vi "G#RemoteProxy_Create.vi"(0 "reference in":refnum<class "G#RemoteProxy.lvclass">, 1 "proxy class ref":refnum<class "G#RemoteProxy.lvclass">, 2 "object name":string, 3 "class name":string, 4 "lvlib hierarchy":string[](array[string]), 5 "full class name":string, 6 "no registration (F)":bool, 7 "error in (no error)":errorcluster, 8 "create method":T3=enum."Create or look up existing", 9 "user counter (T)?":bool=TRUE, 10 "remote object ref":refnum<class "G#Object.lvclass">, 11 "class hierarchy":T2[](array[typedef]), 12 "connection ID":refnum<k5>, 13 "id":u32, 14 "address":u32, 15 "owner":string, 17 "in memory?":bool) -> (20 "reference out":refnum<class "G#RemoteProxy.lvclass">, 23 "# of users":i32, 27 "error out":errorcluster)   [LabVIEW 2017, in "G#RemoteProxy.lvclass"]
doc: "Constructor."
uses:
  <vilib>/addons/_AddQ/G#Debugger/G#RemoteProxy/G#RemoteProxy.lvclass
  C:/Program Files (x86)/National Instruments/LabVIEW 2017/vi.lib/addons/_AddQ/G#Object/G#Object.lvclass
  <vilib>/addons/_AddQ/G#Object/utils/G#Object_CreateMethod.ctl
  <vilib>/addons/_AddQ/G#Object/utils/G#Object_ClassHierarchy.ctl
  <vilib>/addons/_AddQ/G#Debugger/G#RemoteProxy/protected/ObjectAttributesProxy.ctl
  <vilib>/addons/_AddQ/G#Object/G#Object.lvclass
  <vilib>/addons/_AddQ/G#Debugger/G#RemoteProxy/G#RemoteProxy.lvclass/G#RemoteProxy.ctl
panel:
  in  "object attributes type":T1
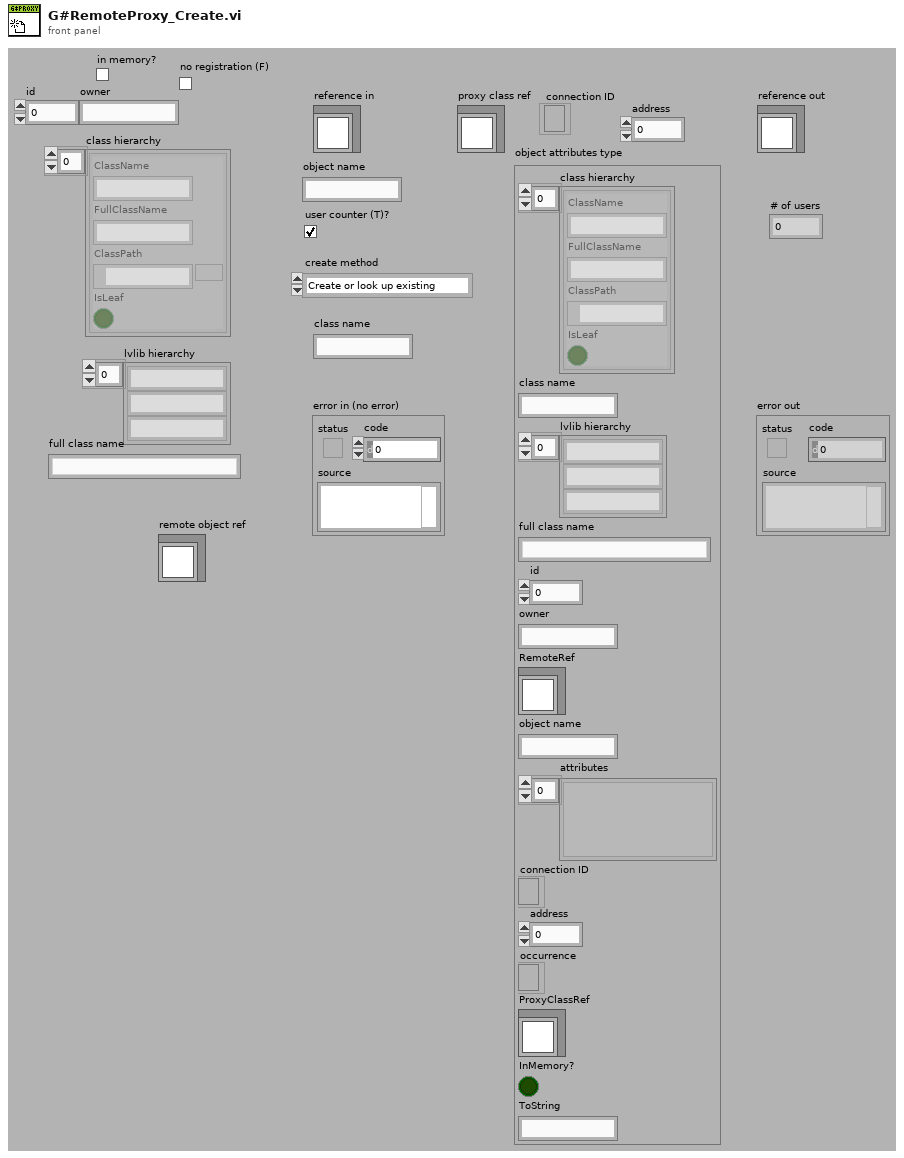
[diagram p1: front panel]
types:
  T1 = typedef "G#RemoteProxy.lvclass/ObjectAttributesProxy.ctl" = cluster{"class hierarchy":T2[], "class name":string, "lvlib hierarchy":string[], "full class name":string, "id":u32, "owner":string, "RemoteRef":refnum<class "G#Object.lvclass">, "object name":string, "attributes":variant[], "connection ID":refnum<k5>, "address":u32, "occurrence":refnum<k4>, "ProxyClassRef":refnum<class "G#RemoteProxy.lvclass">, "InMemory?":bool, "ToString":string}
  T2 = typedef "G#Object.lvclass/G#Object_ClassHierarchy.ctl" = cluster{"ClassName":string, "FullClassName":string, "ClassPath":path, "IsLeaf":bool}
  T3 = typedef "G#Object.lvclass/G#Object_CreateMethod.ctl" = enum16{"Create", "Create or look up existing", "Look up existing"}
  T4 = typedef "G#RemoteProxy.lvclass/ObjectAttributesRef.ctl" = refnum<data-value>
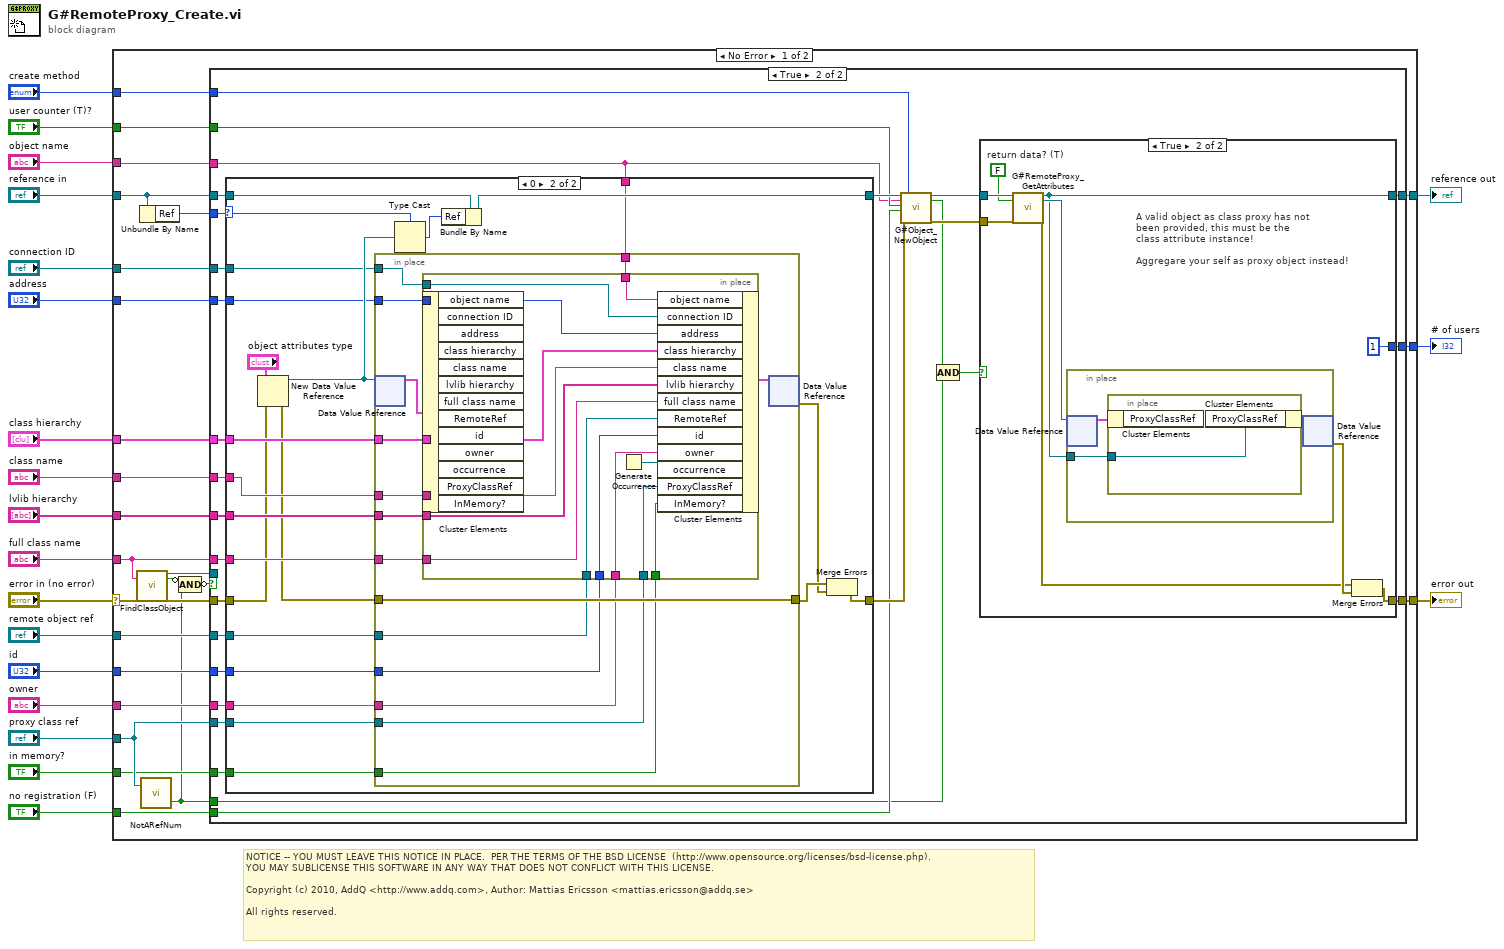
[diagram p0: block diagram]
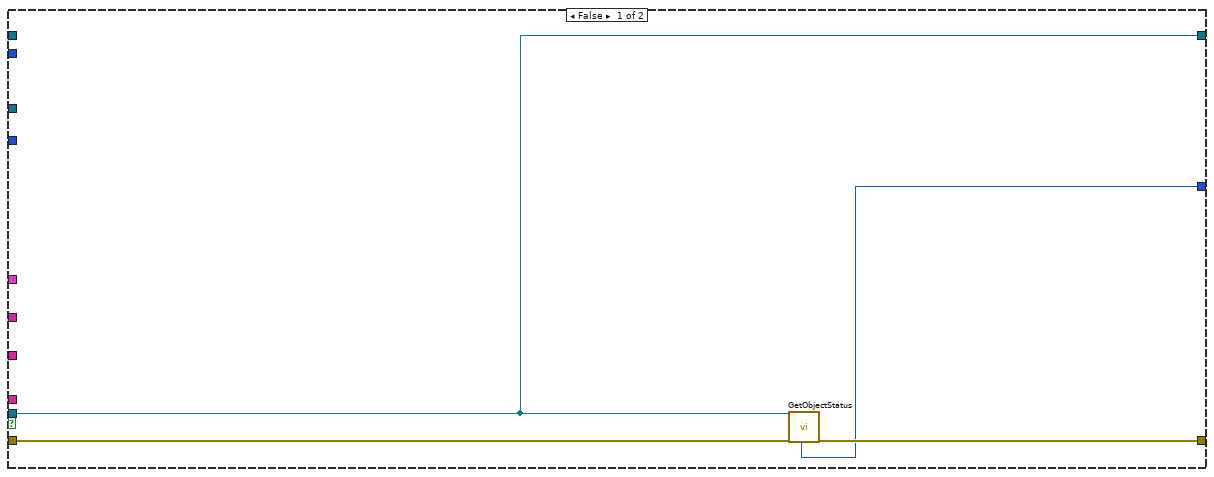
[diagram p2: hidden frame]
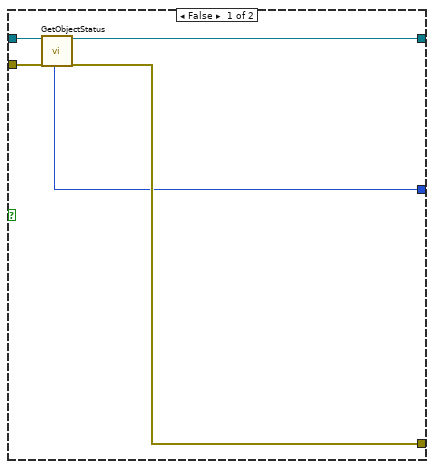
[diagram p3: hidden frame]
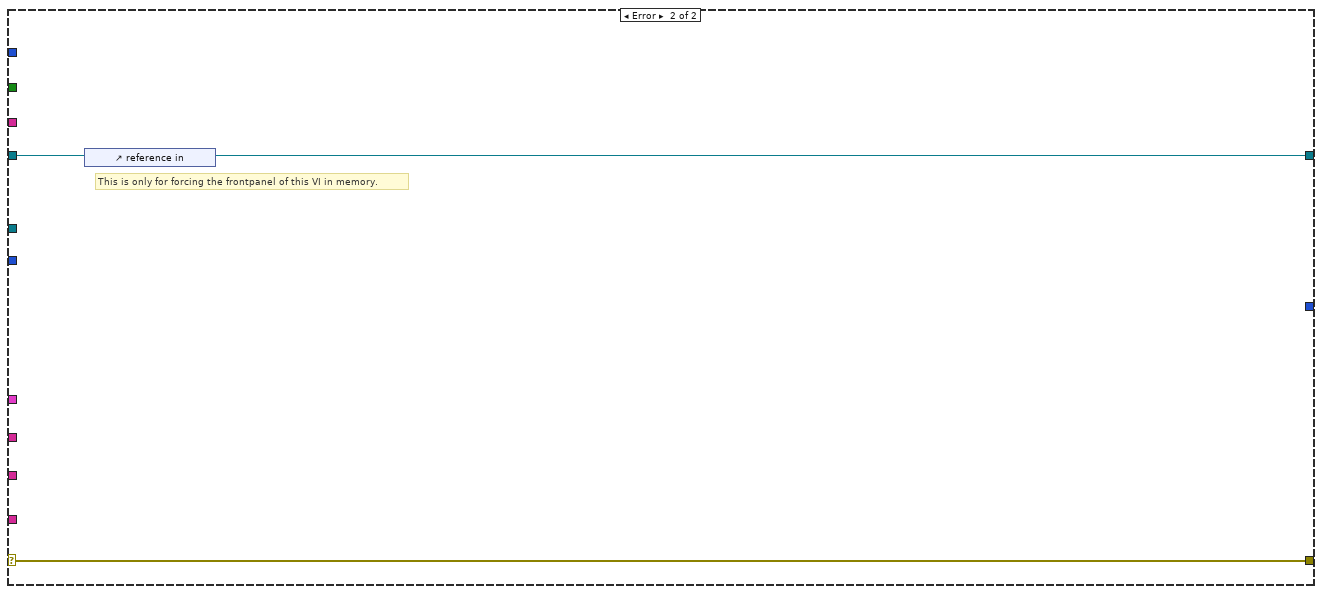
[diagram p5: hidden frame]
diagram:
  # "NOTICE -- YOU MUST LEAVE THIS NOTICE IN PLACE.  PER THE TERMS OF THE BSD LICENSE  (http://www.opensource.org/licenses/bsd-license.php).\nYOU MAY SUBLICENSE THIS SOFTWARE IN ANY WAY THAT DOES NOT CONFLICT WITH THIS LICENSE.\n\nCopyright (c) 2010, AddQ <http://www.addq.com>, Author: Mattias Ericsson <mattias.ericsson@addq.se>\n\nAll rights reserved."
  n1 = case shown="No Error" "error in (no error)" {
    selector: "error in (no error)" -> [w29 w151]
    tunnel: [w33 w151] -> w19
    tunnel: [w32 w150] -> w17
    tunnel: "reference in" -> [w26 w150]
    tunnel: "create method" -> [w43 _]
    tunnel: "object name" -> [w38 _]
    tunnel: "user counter (T)?" -> [w42 _]
    tunnel: "class hierarchy" -> [w46 _]
    tunnel: "class name" -> [w45 _]
    tunnel: "lvlib hierarchy" -> [w44 _]
    tunnel: "full class name" -> [w27 _]
    tunnel: "remote object ref" -> [w41 _]
    tunnel: "id" -> [w40 _]
    tunnel: "owner" -> [w39 _]
    tunnel: "connection ID" -> [w37 _]
    tunnel: "address" -> [w36 _]
    tunnel: "no registration (F)" -> [w35 _]
    tunnel: "proxy class ref" -> [w34 _]
    tunnel: [w31 _] -> w2
    tunnel: "in memory?" -> [w30 _]
    frame No Error {
      n2 = call <vilib>:"FindClassObject.vi"("full class name"=w27, "error in (no error)"=w29) -> ("proxy class object ref"=w21:refnum<class "G#RemoteProxy.lvclass">, "not found?"=w23:bool, "error out"=w28:errorcluster)  [unwired: 15 in]
      n3 = Unbundle By Name(w26) -> ("Ref"=w25:u32)
      n4 = call-dynamic "NotARefNum.vi"("reference in"=w34) -> ("not a refnum?"=w24:bool)  [unwired: 1 in, 1 out]
      n5 = Compound Arithmetic op=AND(invert w23, w24) -> (invert w22:bool)
      n6 = case shown="True" w22 {
        tunnel: w46 -> [_ w78]
        tunnel: w45 -> [_ w77]
        tunnel: w44 -> [_ w76]
        tunnel: w26 -> [_ w52]
        tunnel: w43 -> [_ w73]
        tunnel: w42 -> [_ w72]
        tunnel: w41 -> [_ w71]
        tunnel: w40 -> [_ w70]
        tunnel: w39 -> [_ w69]
        tunnel: w38 -> [_ w68]
        tunnel: w37 -> [_ w67]
        tunnel: w36 -> [_ w66]
        tunnel: w35 -> [_ w65]
        tunnel: w34 -> [_ w64]
        tunnel: [w49 w63] -> w33
        tunnel: [w48 w61] -> w32
        tunnel: w24 -> [_ w57]
        tunnel: [w47 w56] -> w31
        tunnel: w30 -> [_ w55]
        tunnel: w28 -> [w50 w54]
        tunnel: w27 -> [_ w53]
        tunnel: w25 -> [_ w51]
        tunnel: w21 -> [w48 _]
        frame False {
          n7 = call-dynamic "GetObjectStatus.vi"("reference in"=w48, "error in (no error)"=w50) -> ("# of users?"=w47:i32, "error out"=w49:errorcluster)  [unwired: 6 in, 10 out]
        }
        frame True {
          n8 = case shown="0" w51 {
            selector: w51 -> [_ w103]
            tunnel: w78 -> [_ w119]
            tunnel: w77 -> [_ w118]
            tunnel: w76 -> [_ w117]
            tunnel: w53 -> [_ w116]
            tunnel: w54 -> [w97 w114]
            tunnel: w52 -> [w98 w112]
            tunnel: [w97 w109] -> w75
            tunnel: [w98 w108] -> w74
            tunnel: w71 -> [_ w107]
            tunnel: w70 -> [_ w106]
            tunnel: w69 -> [_ w105]
            tunnel: w68 -> [_ w104]
            tunnel: w67 -> [_ w102]
            tunnel: w66 -> [_ w101]
            tunnel: w64 -> [_ w100]
            tunnel: w55 -> [_ w99]
            frame Default {
              # "Already created"
            }
            frame 0 {
              n9 = New Data Value Reference(data value="object attributes type", error in=w114) -> (data value reference=w110:refnum<data-value>, error out=w113:errorcluster)
              n10 = in-place {
                in-place-border: w113 -> [w134]
                in-place-border: [w134] -> w121
                in-place-border: w119 -> [w133]
                in-place-border: w118 -> [w132]
                in-place-border: w117 -> [w131]
                in-place-border: w116 -> [w130]
                in-place-border: w107 -> [w129]
                in-place-border: w106 -> [w128]
                in-place-border: w105 -> [w127]
                in-place-border: w104 -> [w126]
                in-place-border: w102 -> [w125]
                in-place-border: w101 -> [w124]
                in-place-border: w100 -> [w123]
                in-place-border: w99 -> [w122]
                n11 = in-place-dvr #1(w110) -> (w135:T1)  [unwired: 1 out]
                n12 = in-place {
                  in-place-border: w133 -> [w149]
                  in-place-border: w132 -> [w148]
                  in-place-border: w131 -> [w147]
                  in-place-border: w130 -> [w146]
                  in-place-border: w129 -> [w145]
                  in-place-border: w128 -> [w144]
                  in-place-border: w127 -> [w143]
                  in-place-border: w126 -> [w141]
                  in-place-border: w125 -> [w142]
                  in-place-border: w124 -> [w140]
                  in-place-border: w123 -> [w138]
                  in-place-border: w122 -> [w137]
                  n13 = in-place-cluster #2(w135) -> ()  [unwired: 13 out]
                  n14 = Generate Occurrence() -> (w139:refnum<k4>)
                  n15 = in-place-cluster #2("object name"=w141, "connection ID"=w142, "address"=w140, "class hierarchy"=w149, "class name"=w148, "lvlib hierarchy"=w147, "full class name"=w146, "RemoteRef"=w145, "id"=w144, "owner"=w143, "occurrence"=w139, "ProxyClassRef"=w138, "InMemory?"=w137) -> (w136:T1)
                }
                n16 = in-place-dvr #1(w136) -> (w120:errorcluster)  [unwired: 1 out]
              }
              n17 = Type Cast(type=w103, x=w110) -> (*(type *) &x=w111:u32)
              n18 = Bundle By Name(cluster=w112, "Ref"=w111) -> (w108:refnum<class "G#RemoteProxy.lvclass">)
              n19 = Merge Errors(w121, w120) -> (w109:errorcluster)
            }
          }
          n20 = call <vilib>:"G#Object_NewObject.vi"("reference in"=w74, "object name (\"\")"=w68, "user counter (T)"=w72, "no registration (F)"=w65, "error in (no error)"=w75, "create method"=w73) -> ("reference out"=w62:refnum<class "G#RemoteProxy.lvclass">, "created new?"=w59:bool, "error out"=w60:errorcluster)  [unwired: 11 in]
          n21 = Compound Arithmetic op=AND(w59, w57) -> (w58:bool)
          n22 = case shown="True" w58 {
            tunnel: [w80 w91] -> w63
            tunnel: w62 -> [w83 w90]
            tunnel: [w81 w85] -> w61
            tunnel: w60 -> [w82 w89]
            tunnel: [w79 1 ("# of users?")] -> w56
            frame False {
              n23 = call-dynamic "GetObjectStatus.vi"("reference in"=w83, "error in (no error)"=w82) -> ("# of users?"=w79:i32, "reference out"=w81:refnum<class "G#RemoteProxy.lvclass">, "error out"=w80:errorcluster)  [unwired: 6 in, 9 out]
            }
            frame True {
              w86 = FALSE  # return data? (T)
              # "A valid object as class proxy has not\nbeen provided, this must be the\nclass attribute instance!\n\nAggregare your self as proxy object instead!"
              n24 = call <vilib>:"G#RemoteProxy_GetAttributes.vi"("reference in"=w90, "return data? (T)"=w86, "error in (no error)"=w89) -> ("reference out"=w85:refnum<class "G#RemoteProxy.lvclass">, "attributes ref"=w87:T4, "error out"=w88:errorcluster)  [unwired: 13 in, 1 out]
              n25 = in-place {
                in-place-border: w85 -> [w93]
                n26 = in-place-dvr #3(w87) -> (w94:T1)  [unwired: 1 out]
                n27 = in-place {
                  in-place-border: w93 -> [w96]
                  n28 = in-place-cluster #4(w94) -> ()  [unwired: 1 out]
                  n29 = in-place-cluster #4("ProxyClassRef"=w96) -> (w95:T1)
                }
                n30 = in-place-dvr #3(w95) -> (w92:errorcluster)  [unwired: 1 out]
              }
              n31 = Merge Errors(w88, w92) -> (w91:errorcluster)
            }
          }
        }
      }
    }
    frame Error {
      # "This is only for forcing the frontpanel of this VI in memory."
      n32 = control-ref of="reference in"() -> ()  [unwired: 1 out]
    }
  }
  "error out" <- w19
  "reference out" <- w17
  "# of users" <- w2
